vi "Customized Fixed-Point Filter Modeling and Simulation.vi"() -> ()   [LabVIEW 2023]
doc: "Demonstrates how to use the DFD FXP Set Quantizer VI to customize a fixed-point filter model after you obtain the default model using the DFD FXP Modeling VI.\n\nComplete the following steps to use this VI.\n1) Run the VI.\n2) Select <B>Random Noise</B> from the <B>Source</B> pull-down menu.\n3) Observe the feedback information in the Text Filtering Report.\n4) Observe the mean squared error (MSE) value to compare the fixed-point filtering result with the floating-point filtering result.\n5) Observe the <B>Fixed-Point Model</B> input for information about the default fixed-point model that you obtained by using the DFD FXP Modeling VI.\n5) Modify the <B>wl</B> setting of the Multiplicand quantizer and view the effect on the MSE value.\n6) Click the <B>STOP</B> button to stop this VI.\n7) Examine the block diagram to learn the importance of quantizing the input signal before feeding the input signal into floating-point filtering block."
uses:
  <vilib>/addons/Digital Filter Design/_Objects.llb/DFD Quantization Settings.ctl
  <vilib>/addons/Digital Filter Design/_Objects.llb/DFD Quantization Sources.ctl
  <vilib>/addons/Digital Filter Design/_Objects.llb/DFD FXP Statistics Data.ctl
  <vilib>/addons/Digital Filter Design/FXPModel.llb/DFD FXP Quantize Coef (Easy).vi
  <vilib>/addons/Digital Filter Design/FXPModel.llb/DFD FXP Get Quantizer (All).vi
  <vilib>/addons/Digital Filter Design/FXPModel.llb/DFD FXP Set Quantizer (Group).vi
  <vilib>/addons/Digital Filter Design/FXPModel.llb/DFD FXP Get Quantizer (One).vi
  <vilib>/Utility/VariantDataType/GetNumericFxpInfo.vi
  <vilib>/addons/Digital Filter Design/FXPSim.llb/dfd_Check Input FXP Settings.vi
  <vilib>/addons/Digital Filter Design/FXPSim.llb/dfd_Check SRate Simulation Integer Input.vi
  <vilib>/addons/Digital Filter Design/FXPSim.llb/dfd_FXP Simu.vi
  <vilib>/addons/Digital Filter Design/Process.llb/DFD Filtering (Array).vi
  <vilib>/addons/Digital Filter Design/FXPSim.llb/SimXnode/DFD FXP Simulation.xnode
  <vilib>/addons/Digital Filter Design/_Objects.llb/DFD Filter Obj.ctl
  <vilib>/addons/Digital Filter Design/_Objects.llb/DFD Filter Coef.ctl
  <vilib>/addons/Digital Filter Design/_Objects.llb/DFD Filter Structure Type Selector.ctl
  <vilib>/addons/Digital Filter Design/_Objects.llb/dfd_Internal Quantization Settings.ctl
  <vilib>/addons/Digital Filter Design/_Objects.llb/dfd_Internal Quantization Srcs.ctl
  <vilib>/addons/Digital Filter Design/_Objects.llb/DFD Coef Norm Type.ctl
  <vilib>/Analysis/NI_AALBase.lvlib
  <vilib>/addons/Digital Filter Design/NI_DigFilterLicensed.lvlib
  <vilib>/Analysis/NI_AALPro.lvlib
  <vilib>/addons/Digital Filter Design/NI_DigFilter_FXP.lvlib
  <vilib>/Utility/VariantDataType/VariantType.lvlib
panel:
  out "MSE":dbl format="%.6g"
  in  "Output Word Length":i16=16
  in  "Input Word Length":i16=16
  in  "Source":enum16{"Sine", "Random Noise"}(ring)
  in  "Number of Samples":i32=128
  in  "stop":bool
  out "Filtering Text Report":string
  out "Filtered Signals":dbl[][](graph)
  in  "Fixed-Point Model":T1[](array[typedef])=[{"source"=1, "wl"=16, "iwl"=1, "overflow mode"=enum."Saturation", "rounding mode"=enum."Truncation", "signed?"=TRUE}, {"source"=2, "wl"=16, "iwl"=1, "overflow mode"=enum."Saturation", "rounding mode"=enum."Truncation", "signed?"=TRUE}, {"source"=3, "wl"=16, "iwl"=1, "overflow mode"=enum."Wrap", "rounding mode"=enum."Truncation", "signed?"=TRUE}, {"source"=4, "wl"=32, "iwl"=2, "overflow mode"=enum."Wrap", "rounding mode"=enum."Truncation", "signed?"=TRUE}, {"source"=5, "wl"=32, "iwl"=2, "overflow mode"=enum."Wrap", "rounding mode"=enum."Truncation", "signed?"=TRUE}, {"source"=6, "wl"=16, "iwl"=1, "overflow mode"=enum."Wrap", "rounding mode"=enum."Truncation", "signed?"=TRUE}] {"source" items=["Coefficients a/k"=0, "Coefficients b/v"=7, "Input"=1, "Output"=2, "Multiplicand"=3, "Product"=4, "Sum"=5, "Delay"=6]}
  # "Select Help>>Show Context Help and move the cursor over the VI icon for more information."
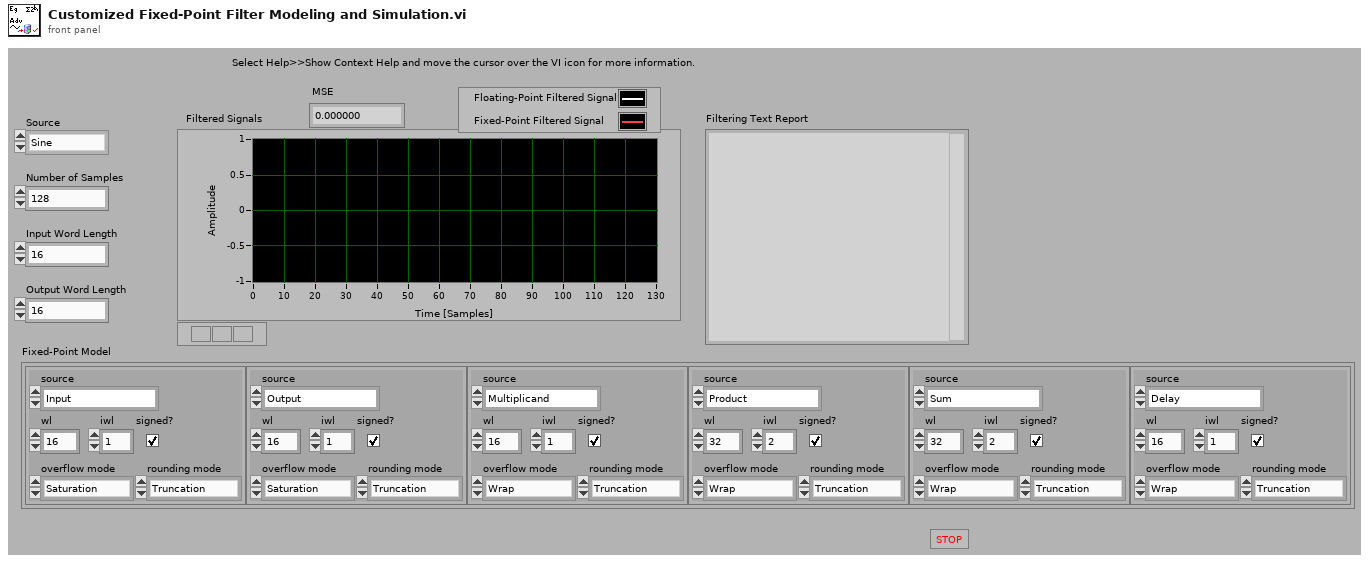
[diagram p1: front panel]
types:
  T1 = typedef "NI_DigFilterLicensed.lvlib/DFD Quantization Settings.ctl" = cluster{"source":T2, "wl":i16, "iwl":i16, "overflow mode":enum16{"Saturation", "Wrap"}, "rounding mode":enum16{"Nearest", "Truncation"}, "signed?":bool}
  T2 = typedef "NI_DigFilterLicensed.lvlib/DFD Quantization Sources.ctl" = u16
  T3 = typedef "NI_DigFilterLicensed.lvlib/DFD FXP Statistics Data.ctl" = cluster{"max value":ext, "min value":ext, "#overflows":i32, "#underflows":i32, "#operations":i32}
  T4 = cluster{"quantizer source":T2, "statistical information":T3}[]
  T5 = typedef "NI_DigFilterLicensed.lvlib/DFD Filter Obj.ctl" = cluster{"mSRate_Fs":dbl, "mSRate_Version":string, "mSRate_Comments":string, "mSRate_OrgCoef":T6, "mSRate_CurCoef":T6, "mSRate_Quantized?":bool, "mSRate_QCoef":T6, "mSRate_QSettings":T8[], "mSRate_Order":i32, "mSRate_Scaling":cluster{"mSRate_ScaleByPowerOf2?":bool, "mSRate_ScaleType":T10}}
  T6 = typedef "NI_DigFilterLicensed.lvlib/DFD Filter Coef.ctl" = cluster{"type":T7, "gain":dbl, "coef a (k)":dbl[], "coef b (v)":dbl[]}
  T7 = typedef "NI_DigFilterLicensed.lvlib/DFD Filter Structure Type Selector.ctl" = enum16{"Undefined", "FIR Direct Form", "FIR Direct Form Transposed", "FIR Symmetric", "FIR Antisymmetric", "IIR Direct Form I", "IIR Direct Form I Transposed", "IIR Direct Form II", "IIR Direct Form II Transposed", "IIR Cascaded Second Order Sections Form I", "IIR Cascaded Second Order Sections Form I Transposed", "IIR Cascaded Second Order Sections Form II", "IIR Cascaded Second Order Sections Form II Transposed", "Lattice Allpass (basic sections)", "Lattice Allpass (one multiplier sections)", "Lattice Allpass (normalized sections)", "Lattice AR (basic sections)", "Lattice AR (one multiplier sections)", "Lattice AR (normalized sections)", "Lattice MA (minimum phase)", "Lattice MA (maximum phase)", "Lattice ARMA (basic sections)", "Lattice ARMA (one multiplier sections)", "Lattice ARMA (normalized sections)"}
  T8 = typedef "NI_DigFilterLicensed.lvlib/dfd_Internal Quantization Settings.ctl" = cluster{"source":T9, "wl":i16, "iwl":i16, "overflow mode":enum16{"Saturation", "Wrap"}, "rounding mode":enum16{"Nearest", "Truncation"}, "signed?":bool}
  T9 = typedef "NI_DigFilterLicensed.lvlib/dfd_Internal Quantization Srcs.ctl" = u16
  T10 = typedef "NI_DigFilterLicensed.lvlib/DFD Coef Norm Type.ctl" = enum16{"No Norm", "Time Domain 1-Norm", "Time Domain 2-Norm", "Time Domain Inf-Norm"}
  T11 = cluster{"quantizer source":T2, "statistics information":T3}[]
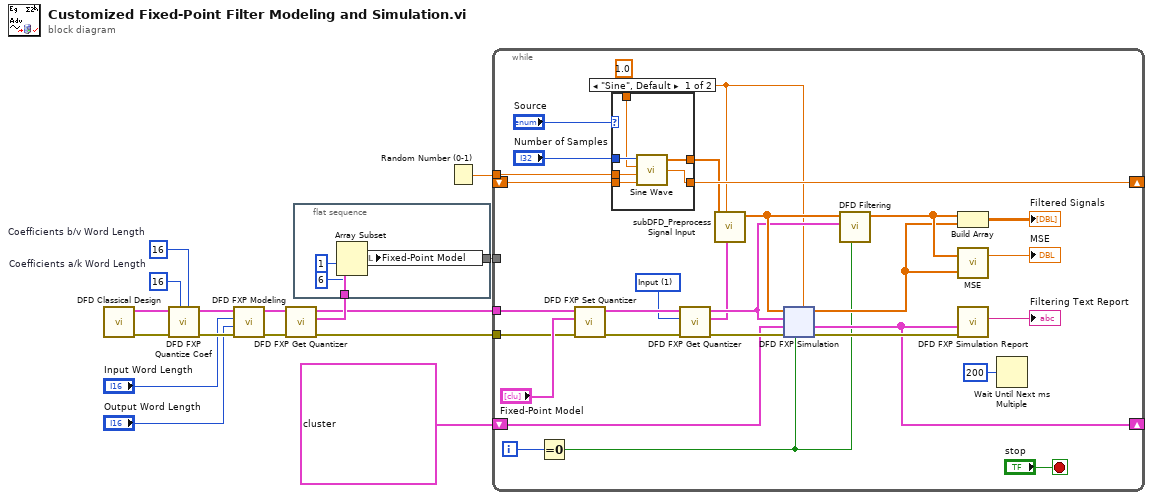
[diagram p0: block diagram]
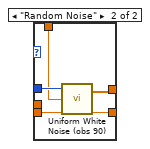
[diagram p2: hidden frame]
diagram:
  w2 = i16 16  # Coefficients b/v Word Length
  w3 = i16 16  # Coefficients a/k Word Length
  n1 = call <vilib>:"DFD Classical Design.vi"() -> ("error out"=w15:errorcluster, "filter out"=w16:T5)  [unwired: 6 in, 4 out]
  n2 = call-poly <vilib>:"DFD FXP Quantize Coef.vi"("coefficients b/v word length"=w2, "coefficients a/k word length"=w3, "error in (no error)"=w15, "filter in"=w16) -> ("error out"=w13:errorcluster, "filter out"=w14:T5)  [unwired: 1 in, 5 out]
  n3 = call <vilib>:"DFD FXP Modeling.vi"("error in (no error)"=w13, "output word length"="Output Word Length", "input word length"="Input Word Length", "filter in"=w14) -> ("error out"=w9:errorcluster, "filter out"=w10:T5)  [unwired: 3 in, 3 out]
  n4 = call-poly <vilib>:"DFD FXP Get Quantizer.vi"("error in (no error)"=w9, "filter in"=w10) -> ("error out"=w7:errorcluster, "quantizers"=w8:T1[], "filter out"=w6:T5)  [unwired: 7 out]
  n5 = flat-sequence {
    tunnel: w8 -> [w20]
    tunnel: [w17] -> w5
    frame #0 {
      n6 = Array Subset(array=w20, index=1, length=6) -> (w17:T1[])
      n7 = local write "Fixed-Point Model"(w17) -> ()
    }
  }
  n8 = Random Number (0-1)() -> (number: 0 to 1=w1:dbl)
  n9 = while {
    tunnel: w6 -> [w41]
    tunnel: w7 -> [w40]
    tunnel: w5 -> [_]
    shift-right: [w27] -> _
    shift-left: T4 [{"quantizer source"=1, "statistical information"={"max value"=-inf, "min value"=inf, "#overflows"=0, "#underflows"=0, "#operations"=0}}, {"quantizer source"=2, "statistical information"={"max value"=-inf, "min value"=inf, "#overflows"=0, "#underflows"=0, "#operations"=0}}, {"quantizer source"=3, "statistical information"={"max value"=-inf, "min value"=inf, "#overflows"=0, "#underflows"=0, "#operations"=0}}, {"quantizer source"=4, "statistical information"={"max value"=-inf, "min value"=inf, "#overflows"=0, "#underflows"=0, "#operations"=0}}, {"quantizer source"=5, "statistical information"={"max value"=-inf, "min value"=inf, "#overflows"=0, "#underflows"=0, "#operations"=0}}, {"quantizer source"=6, "statistical information"={"max value"=-inf, "min value"=inf, "#overflows"=0, "#underflows"=0, "#operations"=0}}] ("filtering statistics in") -> [w28]
    shift-right: [w25] -> _
    shift-left: _ -> [w26]
    tunnel: w1 -> [w21]
    i -> [w39]
    stop <- "stop" stop-if-true
    w23 = 1.0 ("amplitude")
    w30 = T2 1 items=["Coefficients a/k"=0, "Coefficients b/v"=7, "Input"=1, "Output"=2, "Multiplicand"=3, "Product"=4, "Sum"=5, "Delay"=6] ("quantizer source")
    n10 = Equal To 0?(x=w39) -> (x = 0?=w22:bool)
    n11 = call-poly <vilib>:"DFD FXP Set Quantizer.vi"("error in (no error)"=w40, "quantizers"="Fixed-Point Model", "filter in"=w41) -> ("error out"=w32:errorcluster, "filter out"=w34:T5)  [unwired: 7 out]
    n12 = case shown="\"Sine\", Default" "Source" {
      tunnel: [w88 w91] -> w24
      tunnel: "Number of Samples" -> [w87 w92]
      tunnel: w26 -> [w86 w90]
      tunnel: [w85 w90] -> w25
      tunnel: w23 -> [w84 w89]
      tunnel: w21 -> [w83 _]
      frame "Sine", Default {
        n13 = call <vilib>:"Sine Wave.vi"("samples"=w87, "amplitude"=w84, "frequency"=w83, "phase in"=w86) -> ("sine wave"=w88:dbl[], "phase out"=w85:dbl)  [unwired: 1 in, 1 out]
      }
      frame "Random Noise" {
        n14 = call <vilib>:"Uniform White Noise (obs 90).vi"("amplitude"=w89, "samples"=w92) -> ("uniform white noise"=w91:dbl[])  [unwired: 1 in, 1 out]
      }
    }
    n15 = call-poly <vilib>:"DFD FXP Get Quantizer.vi"("error in (no error)"=w32, "quantizer source"=w30, "filter in"=w34) -> ("error out"=w31:errorcluster, "quantizer"=w29:T1, "filter out"=w33:T5)  [unwired: 6 out]
    n16 = call <vilib>:"subDFD_Preprocess Signal Input.vi"("input quantizer"=w29, "input range"=w23, "x"=w24) -> ("q[x]"=w35:dbl[])  [unwired: 8 out]
    n17 = xnode "DFD FXP Simulation"("input range"=w23, "init? (T)"=w22, "error in (no error)"=w31, "filtering statistics in"=w28, "filter in"=w33, "signal in"=w35) -> ("error out"=w49:errorcluster, "filtering statistics report"=w27:T11, "DBL signal out"=w37:dbl[])  [unwired: 1 out]
    n18 = call-poly <vilib>:"DFD Filtering.vi"("init? (F)"=w22, "filter"=w33, "signal in"=w35) -> ("signal out"=w38:dbl[])  [unwired: 1 in, 7 out]
    n19 = Build Array(w38, w37) -> (→"Filtered Signals":dbl[][])
    n20 = call <vilib>:"MSE.vi"("X Values"=w37, "Y Values"=w38) -> ("mse"=→"MSE":dbl)  [unwired: 1 out]
    n21 = call <vilib>:"DFD FXP Simulation Report.vi"("error in (no error)"=w49, "filtering statistics report"=w27) -> ("filtering text report"=→"Filtering Text Report":string)  [unwired: 9 out]
    n22 = Wait Until Next ms Multiple(millisecond multiple=u32 200) -> ()  [unwired: 1 out]
  }
